vi "poly_average_ith_value_1d_double_array.vi"(1 "0 indexed? (t)":bool=TRUE, 2 "new array":dbl[](array[numeric]) format="%#_13g", 3 "old array":dbl[](array[numeric]) format="%#_13g", 4 "i":i32) -> (7 "average array":dbl[](array[numeric]))   [LabVIEW 2015]
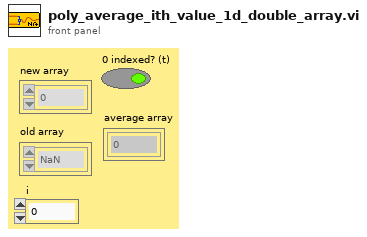
[diagram p1: front panel]
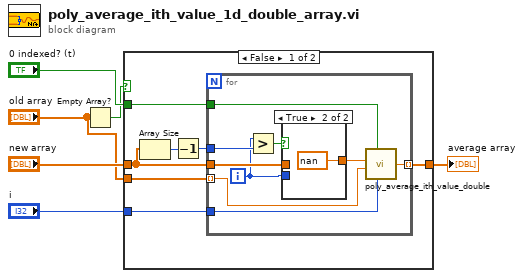
[diagram p0: block diagram]
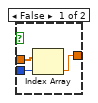
[diagram p2: hidden frame]
diagram:
  n1 = Empty Array?(array="old array") -> (empty?=w1:bool)
  n2 = case shown="False" w1 {
    tunnel: "old array" -> [w13 _]
    tunnel: "new array" -> [w12 w27]
    tunnel: [w9 w27] -> w5
    tunnel: "i" -> [w8 _]
    tunnel: "0 indexed? (t)" -> [w7 _]
    frame False {
      n3 = Array Size(array=w12) -> (size(s)=w11:i32)
      n4 = Decrement(x=w11) -> (x-1=w10:i32)
      n5 = for {
        tunnel: w13 -> [w19] mode=indexing
        tunnel: w12 -> [w22]
        tunnel: w10 -> [w15]
        tunnel: [w18] -> w9 mode=indexing
        tunnel: w8 -> [w17]
        tunnel: w7 -> [w16]
        i -> [w14]
        n6 = Greater?(x=w14, y=w15) -> (0:w21:bool)
        n7 = case shown="True" w21 {
          tunnel: w22 -> [w25 _]
          tunnel: w14 -> [w24 _]
          tunnel: [w23 nan ("new value")] -> w20
          frame False {
            n8 = Index Array(array=w25, index=w24) -> (element=w23:dbl)
          }
          frame True {
          }
        }
        n9 = call "poly_average_ith_value_double.vi"("0 indexed? (T, F = 1 indexed)"=w16, "new value"=w20, "old value"=w19, "i"=w17) -> ("average"=w18:dbl)  [unwired: 4 in]
      }
    }
    frame True {
    }
  }
  "average array" <- w5
